vi "host.vi"() -> ()   [LabVIEW 2012]
panel:
  in  "stop":bool
  out "data":dbl(graph)
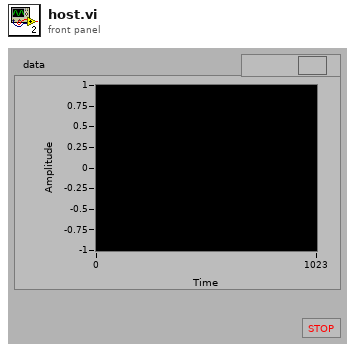
[diagram p1: front panel]
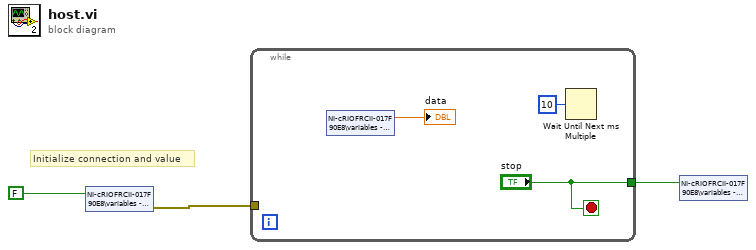
[diagram p0: block diagram]
diagram:
  # "Initialize connection and value"
  n1 = shared-variable "NI-cRIOFRCII-017F90E8\\variables - network - RT.lvlib\\stop"(FALSE) -> (error out=w2:errorcluster)  [unwired: 1 in]
  n2 = while {
    tunnel: ["stop"] -> w3
    tunnel: w2 -> [_]
    stop <- "stop" stop-if-true
    n3 = shared-variable "NI-cRIOFRCII-017F90E8\\variables - network - RT.lvlib\\data"() -> (→"data":dbl)  [unwired: 1 in, 1 out]
    n4 = Wait Until Next ms Multiple(millisecond multiple=u32 10) -> ()  [unwired: 1 out]
  }
  n5 = shared-variable "NI-cRIOFRCII-017F90E8\\variables - network - RT.lvlib\\stop"(w3) -> ()  [unwired: 1 in, 1 out]
